vi "MH_GetWarningsText.vi"(8 "error in (no error)":errorcluster, 10 "warnings":i32, 11 "devidx":i32) -> (0 "error out":errorcluster, 2 "text":string, 3 "return type":i32)   [LabVIEW 2019]
uses:
  MH_DllPath_global.vi
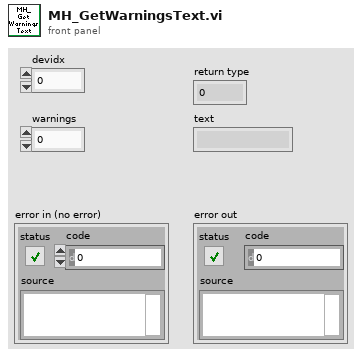
[diagram p1: front panel]
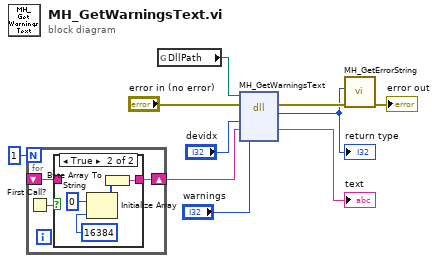
[diagram p0: block diagram]
diagram:
  n1 = for {
    N: 1 -> [_]
    shift-right: [w12] -> w1
    shift-left: _ -> [w11]
    n2 = First Call?() -> (First Call?: T/F=w13:bool)
    n3 = case shown="True" w13 {
      tunnel: [w14 w15] -> w12
      tunnel: w11 -> [w14 _]
      frame False {
      }
      frame True {
        n4 = Initialize Array(u8 0, 16384 ("dimension size")) -> (w16:u8[])
        n5 = Byte Array To String(unsigned byte array=w16) -> (string=w15:string)
      }
    }
  }
  n6 = global read "MH_DllPath_global.vi" "DllPath"() -> (w8:path)
  n7 = dll-call lib="MHLib64.dll" fn="MH_GetWarningsText"(path in=w8, error in="error in (no error)", "devidx"="devidx", "text"=w1, "warnings"="warnings") -> (error out=w7:errorcluster, "return type"=w6:i32, "text"=→"text":string)  [unwired: 3 in, 1 out]
  "return type" <- w6
  n8 = call "MH_GetErrorString.vi"("error in (no error)"=w7, "code"=w6) -> ("error out"=→"error out":errorcluster)  [unwired: 7 in, 2 out]
